vi "Find Next Section_Num-Array-Cluster_.vi"(7 "Min Size":i32=-1, 10 "Find":i32, 11 "Array":cluster{"Array":i32[]}[](array[cluster])) -> (2 "Size Out":i32, 3 "Index":i32, 5 "Array Out":i32[](array[numeric]))   [LabVIEW 2024]
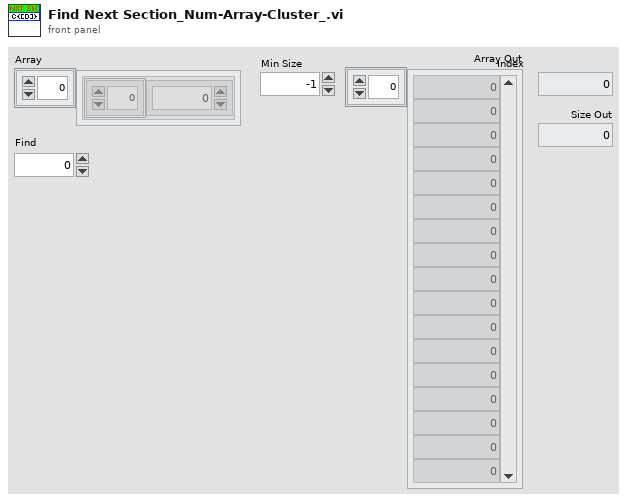
[diagram p1: front panel]
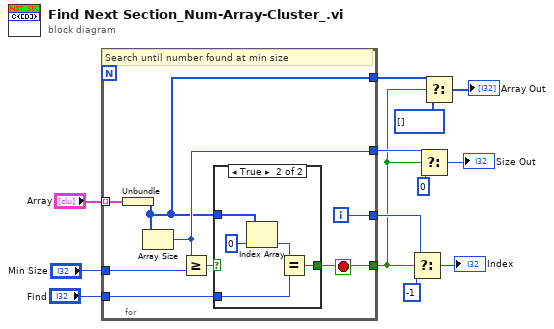
[diagram p0: block diagram]
diagram:
  n1 = for {
    tunnel: "Array" -> [w21] mode=indexing
    tunnel: "Min Size" -> [w20]
    tunnel: "Find" -> [w18]
    tunnel: [w17] -> w10
    tunnel: [w16] -> w3
    tunnel: [w15] -> w7
    tunnel: [w14] -> w4
    i -> [w17]
    stop <- w16 stop-if-true
    # "Search until number found at min size"
    n2 = Unbundle(w21) -> ("Array"=w14:i32[])
    n3 = Array Size(array=w14) -> (size(s)=w15:i32)
    n4 = Greater Or Equal?(x=w15, y=w20) -> (x >= y?=w19:bool)
    n5 = case shown="True" w19 {
      selector: w19 -> [w22 _]
      tunnel: w14 -> [_ w27]
      tunnel: w18 -> [_ w24]
      tunnel: [w22 w23] -> w16
      frame False {
      }
      frame True {
        n6 = Index Array(array=w27, index=0) -> (element=w25:i32)
        n7 = Equal?(x=w25, y=w24) -> (x = y?=w23:bool)
      }
    }
  }
  n8 = Select(t=w10, s=w3, f=-1) -> (s? t:f=→"Index":i32)
  n9 = Select(t=w7, s=w3, f=0) -> (s? t:f=→"Size Out":i32)
  n10 = Select(t=w4, s=w3, f=i32[] [] ("s? t:f")) -> (s? t:f=→"Array Out":i32[])
